vi "Add-element.vi"(8 "error in (no error)":errorcluster, 10 "Elements in":refnum<class "Element-XML.lvclass">[](array[class]), 11 "Element-XML in":refnum<class "Element-XML.lvclass">) -> (0 "error out":errorcluster, 2 "Elements":refnum<class "Element-XML.lvclass">[](array[class]), 3 "Element-XML out":refnum<class "Element-XML.lvclass">)   [LabVIEW 2013, in "MaterialCharacterization.lvlib" / "Element-XML.lvclass"]
uses:
  Element-XML.lvclass
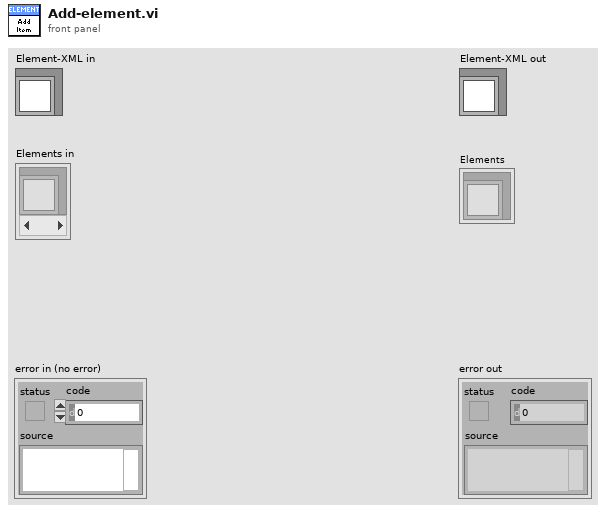
[diagram p1: front panel]
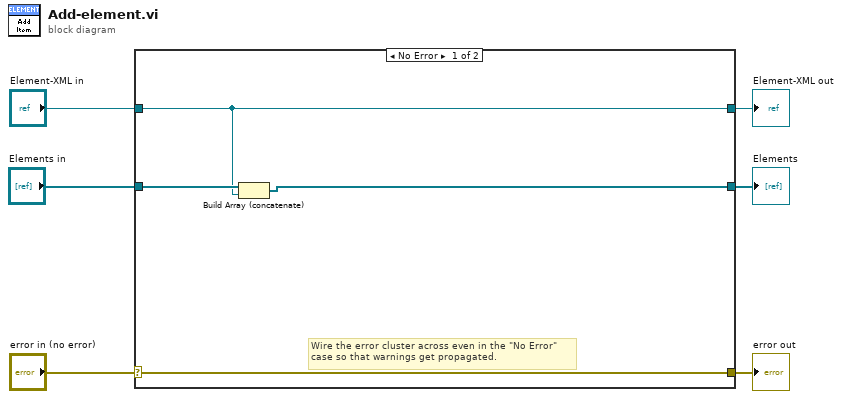
[diagram p0: block diagram]
diagram:
  n1 = case shown="No Error" "error in (no error)" {
    selector: "error in (no error)" -> [w10 w13]
    tunnel: [w10 w13] -> w5
    tunnel: [w8 w12] -> w3
    tunnel: "Element-XML in" -> [w8 w12]
    tunnel: "Elements in" -> [w9 w11]
    tunnel: [w7 w11] -> w1
    frame No Error {
      # "Wire the error cluster across even in the \"No Error\"\ncase so that warnings get propagated."
      n2 = Build Array (concatenate)(w9, w8) -> (w7:refnum<class "Element-XML.lvclass">[])
    }
    frame Error {
    }
  }
  "error out" <- w5
  "Element-XML out" <- w3
  "Elements" <- w1
